vi "7 Hole Probe.vi"() -> (5 "Plug in titles":string[](array[string]), 7 "Plug in values":string[](array[string]))   [LabVIEW 2017]
uses:
  Controls/Inst_type.ctl
  Globals/Meas_global.vi
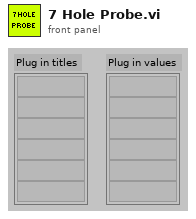
[diagram p1: front panel]
types:
  T1 = typedef "Analysis_info_cluster.ctl" = cluster{"Colour":u32, "Inst type":T2, "Inst name":string, "Symbol":string, "Code name":string, "Extra Info":string, "Inst Array":T3, "Extra Titles":string[], "Extra Values":string[], "U":dbl, "u^2":dbl, "u^3":dbl, "u^4":dbl, "Skew_u":dbl, "Kurt_u":dbl, "Sd Error in Mean":dbl, "% u'/U":dbl, "X":dbl, "Y":dbl, "Z":dbl, "Timescale integral Estimate":dbl, "Sd Error in Variance":dbl, "Calib File":path, "Calib Constants":dbl[], "Output Position":bool, "Full Stats":bool, "Av Sampling Rate":dbl, "Av No of Samples":dbl, "Total Meas Time (s)":dbl, "ADAM Ch Name":string, "Max value":dbl, "Min value":dbl, "Req Sample Rate Hz":dbl, "Sync Delay Time (s)":dbl, "Ch No":i16, "Device ID":string, "Use Latest Calib":bool, "Port":string}
  T2 = typedef "Inst_type.ctl" = enum16{"Propeller anemometer", "Raw voltage", "Pressure Transducer", "Pitot-static tube", "Preston tube", "Hot wire", "Cross wire 1", "Cross wire 2", "Generic Linear", "Generic Polynomial", "Generic BackPoly", "Fast FID", "Thermocouple", "Cold wire", "Pulsed Wire", "LDA Vel", "LDA Tran time", "LDA Arr time", "Microphone"}
  T3 = typedef "Instrument_Array.ctl" = enum16{"PWA", "LDA", "Analogue"}
  T4 = cluster{"Pressure Ch Names":string[], "Pressure Index":i32[], "Metadata Index":i32[], "Port":string}[]
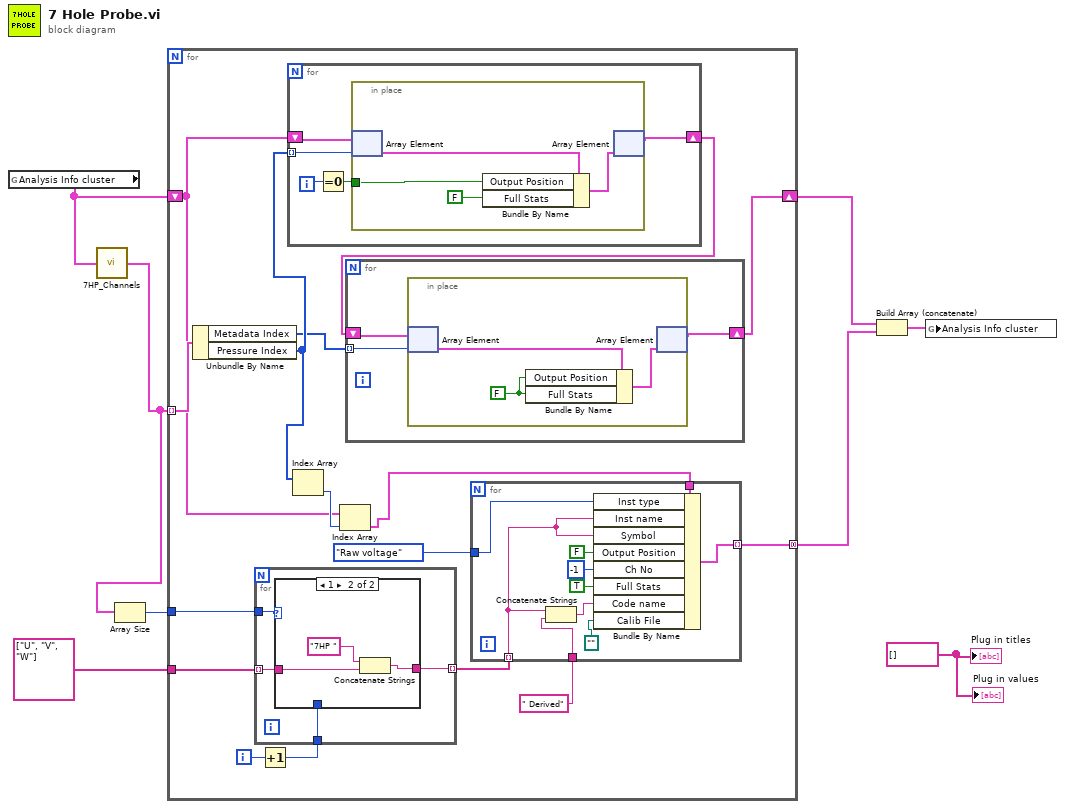
[diagram p0: block diagram]
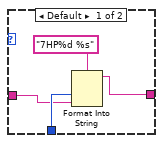
[diagram p2: hidden frame]
diagram:
  w8 = string[] [] ("Plug in titles")
  n1 = global read "Meas_global.vi" "Analysis Info cluster"() -> (w4:T1[])
  n2 = call "7HP_Channels.vi"("Analysis Info cluster"=w4) -> ("7HP Info"=w3:T4)
  n3 = Array Size(array=w3) -> (size(s)=w2:i32)
  n4 = for {
    tunnel: [w23] -> w6 mode=concatenating
    tunnel: w2 -> [w22]
    tunnel: string[] ["U", "V", "W"] ("appended array") -> [w21]
    tunnel: w3 -> [w15] mode=indexing
    shift-right: [w11] -> w1
    shift-left: w4 -> [w13]
    i -> [w19]
    n5 = Unbundle By Name(w15) -> ("Metadata Index"=w10:i32[], "Pressure Index"=w14:i32[])
    n6 = Increment(x=w19) -> (x+1=w18:i32)
    n7 = for {
      tunnel: w22 -> [w43]
      tunnel: w21 -> [w42] mode=indexing
      tunnel: [w41] -> w20 mode=indexing
      tunnel: w18 -> [w40]
      n8 = case shown="1" w43 {
        tunnel: w42 -> [w45 w49]
        tunnel: [w44 w48] -> w41
        tunnel: w40 -> [w46 _]
        frame Default {
          n9 = Format Into String(format string="7HP%d %s", w46, w45) -> (resulting string=w44:string)  [unwired: 2 in, 1 out]
        }
        frame 1 {
          n10 = Concatenate Strings("7HP " ("Inst name"), w49) -> (w48:string)
        }
      }
    }
    n11 = for {
      shift-right: [w31] -> w12
      shift-left: w13 -> [w35]
      tunnel: w14 -> [w34] mode=indexing
      i -> [w33]
      n12 = Equal To 0?(x=w33) -> (x = 0?=w32:bool)
      n13 = in-place {
        in-place-border: w32 -> [w38]
        n14 = in-place-array #1(w35, w34) -> (w37:T1)
        n15 = Bundle By Name(cluster=w37, "Output Position"=w38, "Full Stats"=FALSE) -> (w36:T1)
        n16 = in-place-array #1(w36) -> (w31:T1[])  [unwired: 1 out]
      }
    }
    n17 = Index Array(array=w14) -> (element=w17:i32)  [unwired: 1 in]
    n18 = Index Array(array=w13, index=w17) -> (element=w16:T1)
    n19 = for {
      shift-right: [w25] -> w11
      shift-left: w12 -> [w27]
      tunnel: w10 -> [w26] mode=indexing
      n20 = in-place {
        w28 = FALSE ("Full Stats")
        n21 = in-place-array #2(w27, w26) -> (w30:T1)
        n22 = Bundle By Name(cluster=w30, "Output Position"=w28, "Full Stats"=w28) -> (w29:T1)
        n23 = in-place-array #2(w29) -> (w25:T1[])  [unwired: 1 out]
      }
    }
    n24 = for {
      tunnel: w16 -> [w60]
      tunnel: w20 -> [w54] mode=indexing
      tunnel: [w57] -> w23 mode=indexing
      tunnel: " Derived" -> [w53]
      tunnel: Inst_type."Raw voltage" ("Inst type") -> [w52]
      n25 = Concatenate Strings(w54, w53) -> (w55:string)
      n26 = Bundle By Name(cluster=w60, "Inst type"=w52, "Inst name"=w54, "Symbol"=w54, "Output Position"=FALSE, "Ch No"=i16 -1, "Full Stats"=TRUE, "Code name"=w55, "Calib File"=path "") -> (w57:T1)
    }
  }
  n27 = Build Array (concatenate)(w1, w6) -> (w7:T1[])
  n28 = global write "Meas_global.vi" "Analysis Info cluster"(w7) -> ()
  "Plug in values" <- w8
  "Plug in titles" <- w8
